vi "Host.vi"() -> ()   [LabVIEW 2019]
uses:
  TypeDef/listChannel.ctl
  ByteGSAPIBase/LimsTestStep/acquisitions.ctl
  <vilib>/Bytelabs/ByteChannelsSetting/ChannelSettingsLib/ChannelsRepos/ChannelsRepoXML/ChannelsRepoXML.lvclass
  C:/Program Files (x86)/National Instruments/LabVIEW 2019/vi.lib/Bytelabs/ByteChannelsSetting/ChannelSettingsLib/ChannelsRepos/ChannelsRepoBase/ChannelsRepoBase.lvclass
  TypeDef/TCPMessage.ctl
  <vilib>/Bytelabs/ByteChannelsSetting/ChannelSettingsLib/ChannelsRepos/ChannelsRepoBase/ChannelsRepoBase.lvclass/ChannelsRepoBase.ctl
  TypeDef/ChannelInfo.ctl
  <vilib>/Bytelabs/ByteChannelsSetting/ChannelSettingsLib/ChannelsClasses/ChannelAnalog/AnalogIn/AnalogIn.lvclass
  ByteGSAPIBase/UpdateChannelsList/fields.ctl
  ByteGSAPIBase/TypeDef/Step.ctl
  ByteGSAPIBase/TypeDef/Asset.ctl
  bytetcp/TCPLib/TCP_Class/TCP.lvclass
  <vilib>/Bytelabs/ByteChannelsSetting/ChannelSettingsLib/ChannelsClasses/ChannelBase/ChannelBase.lvclass
  <vilib>/Bytelabs/ByteChannelsSetting/ChannelSettingsLib/ChannelsRepos/ChannelsRepoBase/ChannelsRepoBase.lvclass
  ByteGSAPIBase/ByteGSAPIBase.lvclass
panel:
  in  "Test":T1={"Step Id"=43, "Test Slug"="T0023", "Duration Seconds"=0.0, "Continous?"=FALSE}
  out "error out":errorcluster
  in  "Stop":bool
  out "Results":T2
  in  "Stop Sequence":bool
  out "Status":string
  out "Raws Readings":cluster{"tag":string, "Value":dbl}[](array[cluster])
  in  "Step  Request":bool
  in  "Channel List":T3[](array[typedef])
  in  "Load":bool
  in  "Configuration":bool
  out "Connected?":bool
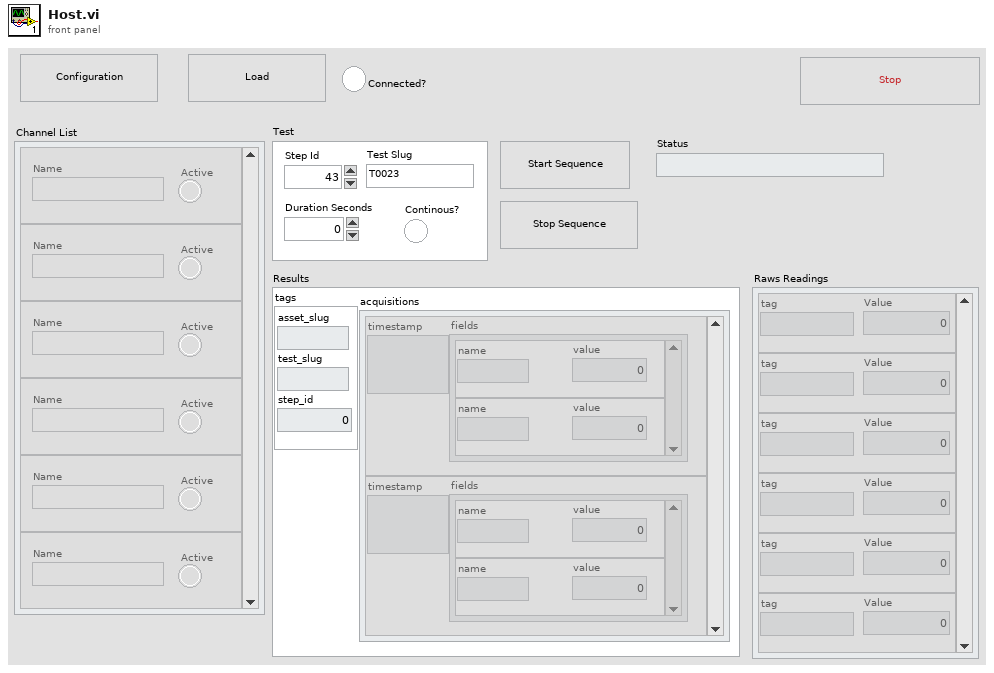
[diagram p1: front panel]
types:
  T1 = cluster{"Step Id":u32, "Test Slug":string, "Duration Seconds":dbl, "Continous?":bool}
  T2 = typedef "ByteGSWebAPI.lvlib/ByteGSAPIBase.lvclass/acquisitions.ctl" = cluster{"tags":cluster{"step_id":i32, "test_slug":string, "asset_slug":string}, "acquisitions":cluster{"timestamp":string, "fields":cluster{"name":string, "value":dbl}[]}[]}
  T3 = typedef "listChannel.ctl" = cluster{"Name":string, "Active":bool}
  T4 = typedef "TCPMessage.ctl" = cluster{"Message":string, "Data":variant}
  T5 = cluster{"Event Registration Refnum":refnum<event-registration>, "ChannelsRepoBase out":refnum<class "ChannelsRepoXML.lvclass">, "TCP_Class":refnum<class "TCP.lvclass">, "Data":variant, "Stauts":string, "notifier out":refnum<notifier>}
  T6 = typedef "ChannelInfo.ctl" = cluster{"Tag":string, "HW Resource":string, "Raw":dbl}
  T7 = typedef "ByteGSWebAPI.lvlib/ByteGSAPIBase.lvclass/fields.ctl" = cluster{"asset_slug":string, "fields":string[]}
  T8 = cluster{"Channel List":T3[], "Test":cluster{"Step Id":u32, "Test Slug":string, "Duration Seconds":dbl, "Continous?":bool}}
  T9 = map{i32, map{string, refnum<class "ChannelBase.lvclass">}}
  T10 = typedef "ByteGSWebAPI.lvlib/ByteGSAPIBase.lvclass/Step.ctl" = cluster{"id":i32, "descrizione":string, "prova":cluster{"slug":string}, "assets":T11[], "criterio_accettazione":string, "valore_criterio_accettazione_max":dbl, "valore_criterio_accettazione_min":dbl, "udm_criterio_accettazione":string, "duration_prova":string, "udm_duration_prova":string, "valore_prova":dbl, "ordine":i32, "user":i32, "link_automation":string, "instruction_automation":string, "data_completamento_checklist":timestamp, "outcome":bool, "step_type":string, "channels":string[]}
  T11 = typedef "ByteGSWebAPI.lvlib/ByteGSAPIBase.lvclass/Asset.ctl" = cluster{"descrizione":string, "slug":string, "id":i32}
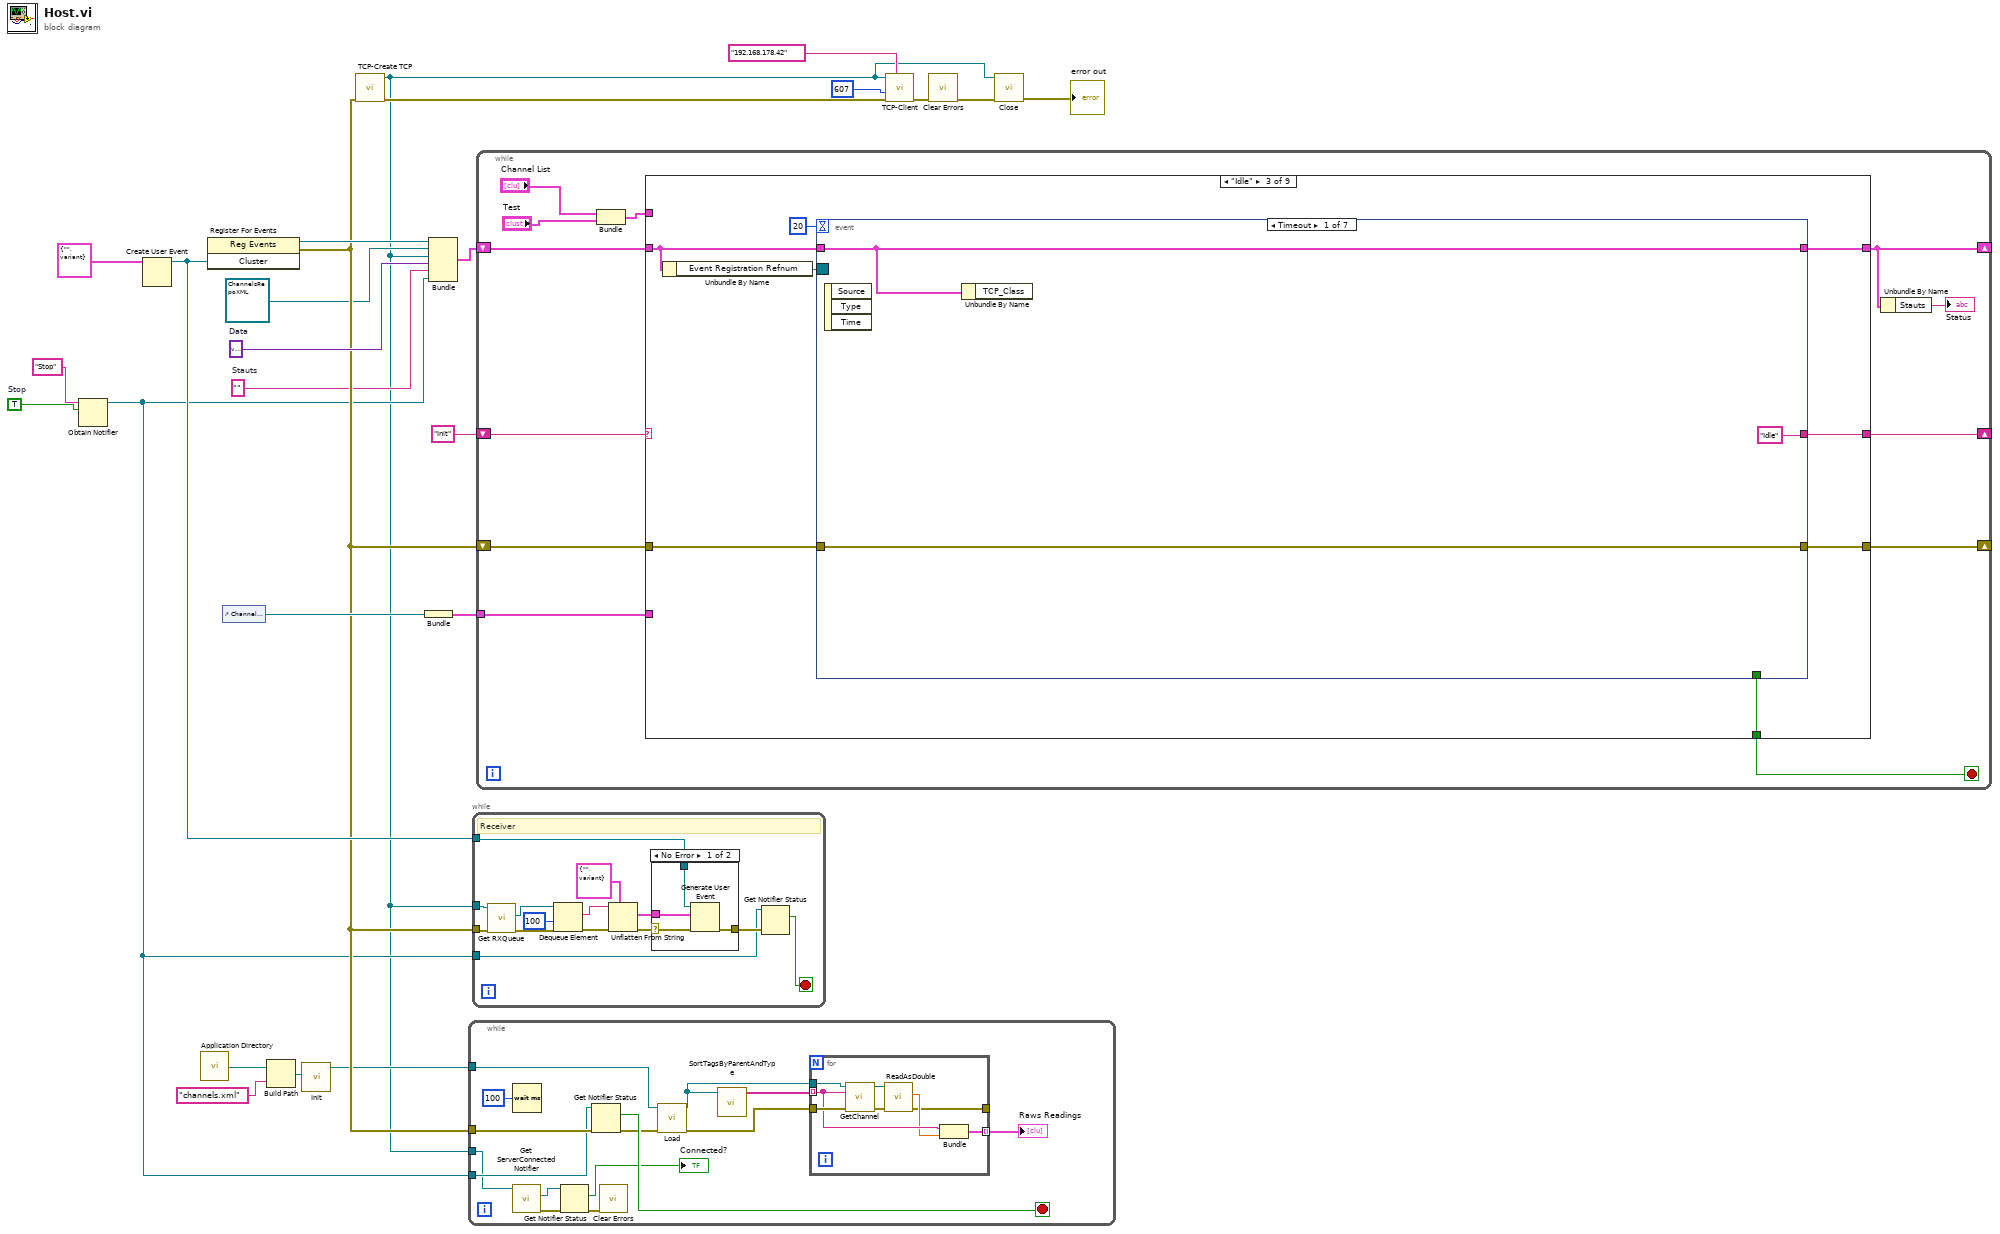
[diagram p0: block diagram]
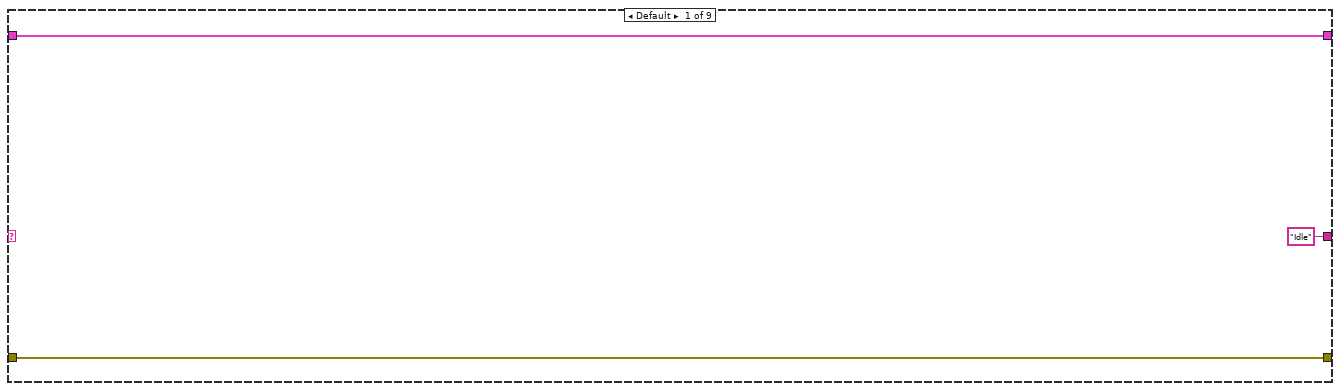
[diagram p2: hidden frame]
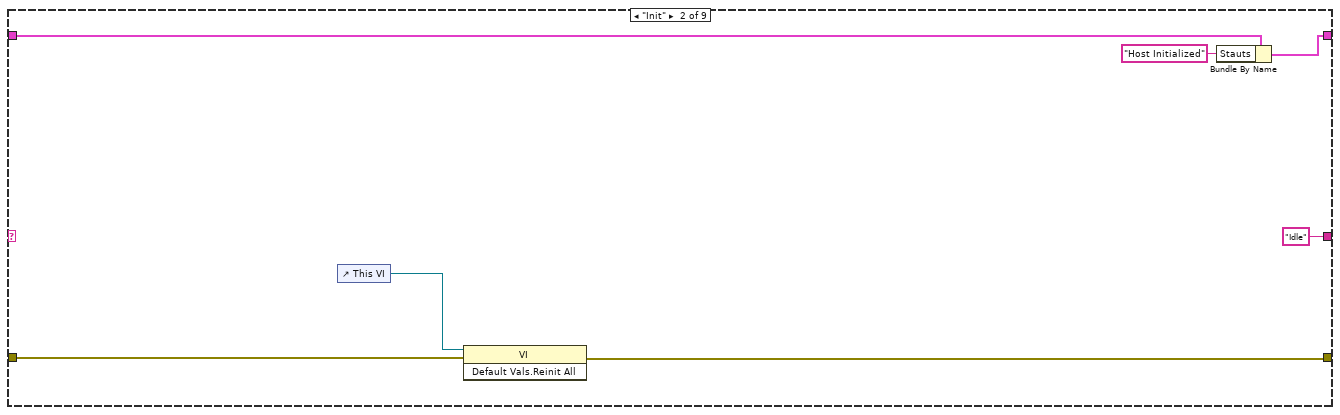
[diagram p3: hidden frame]
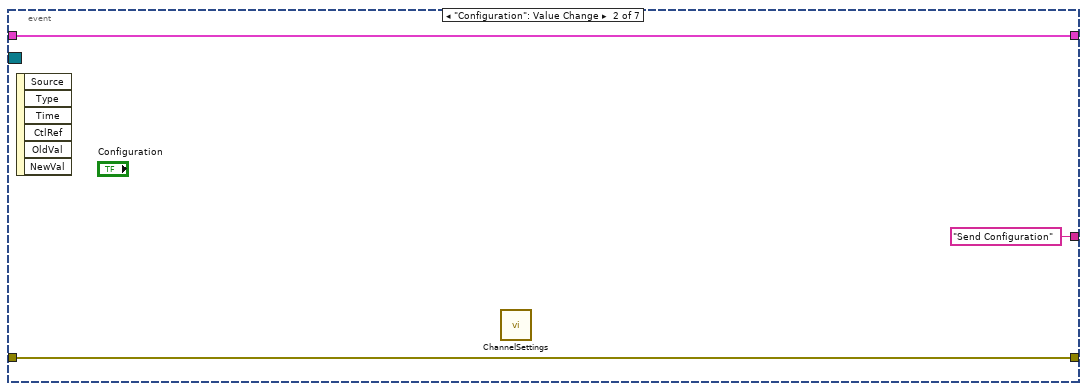
[diagram p4: hidden frame]
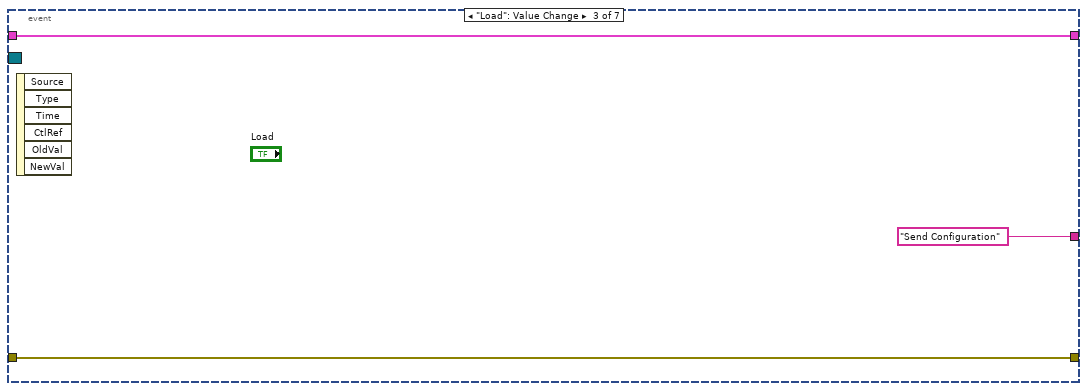
[diagram p5: hidden frame]
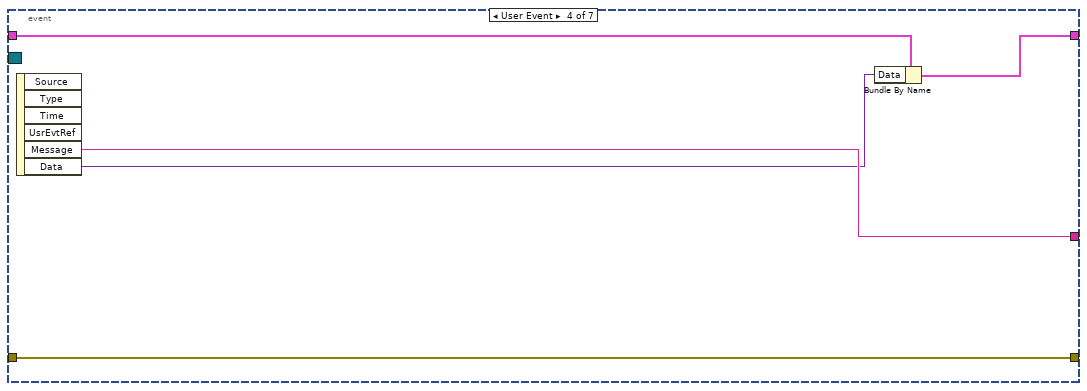
[diagram p6: hidden frame]
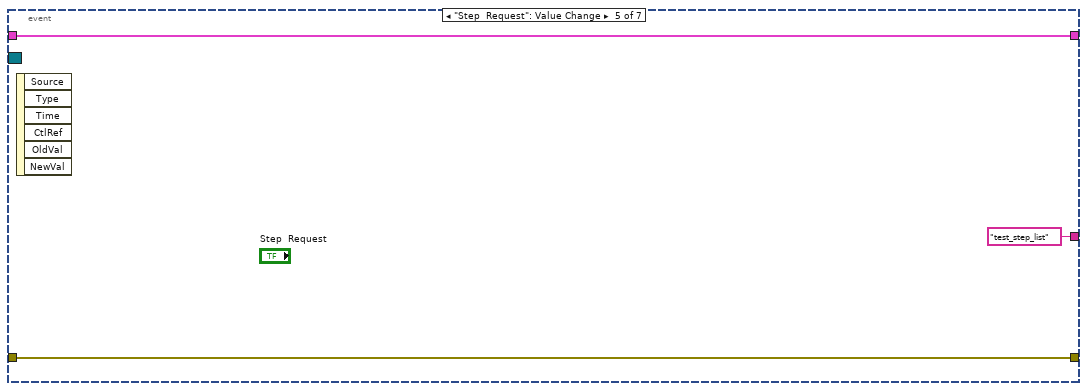
[diagram p7: hidden frame]
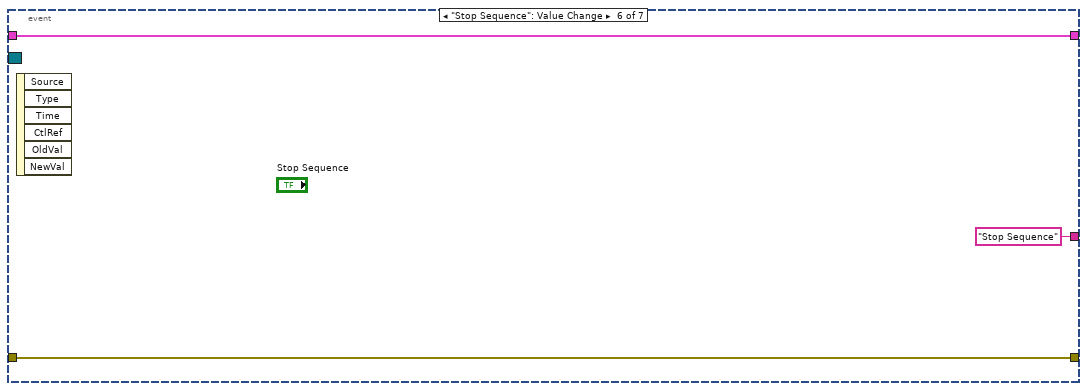
[diagram p8: hidden frame]
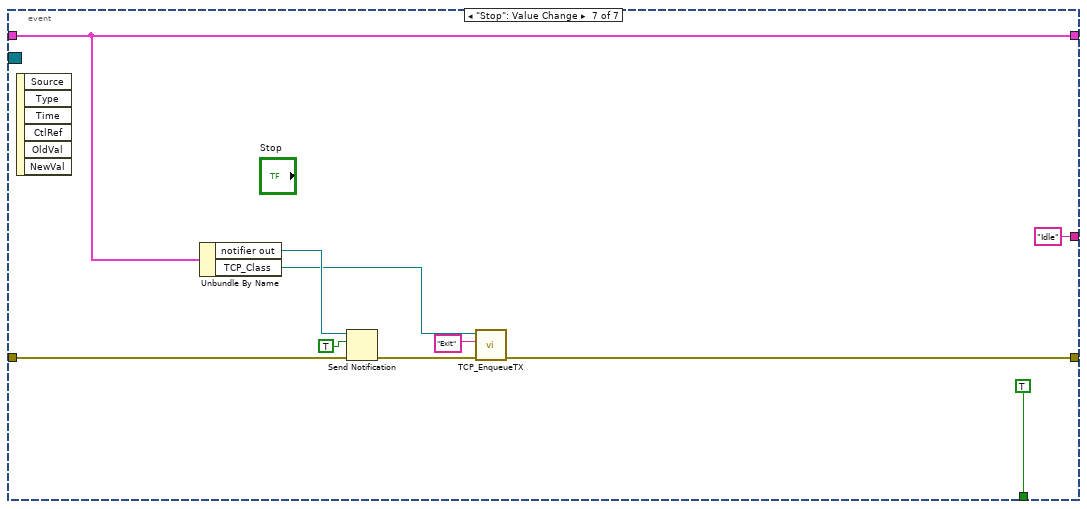
[diagram p9: hidden frame]
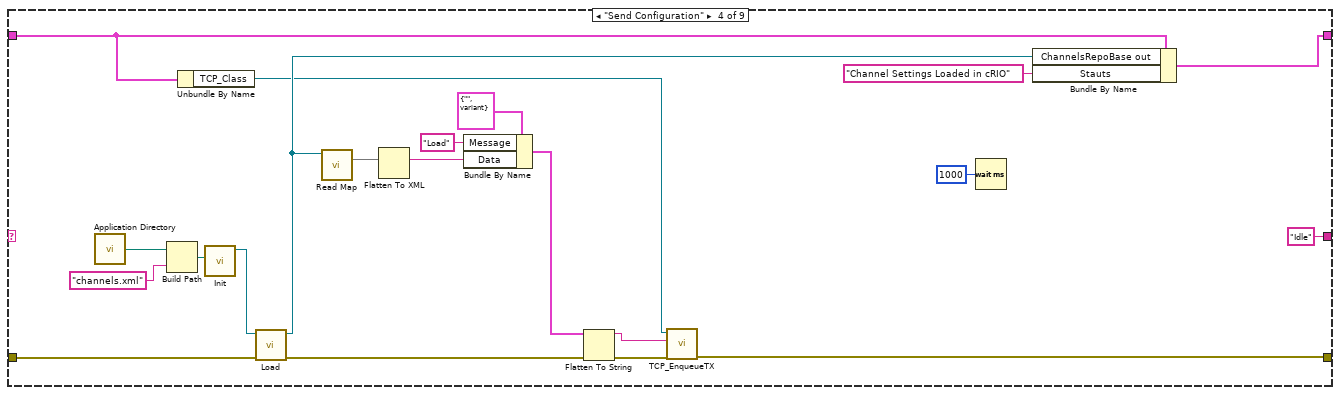
[diagram p10: hidden frame]
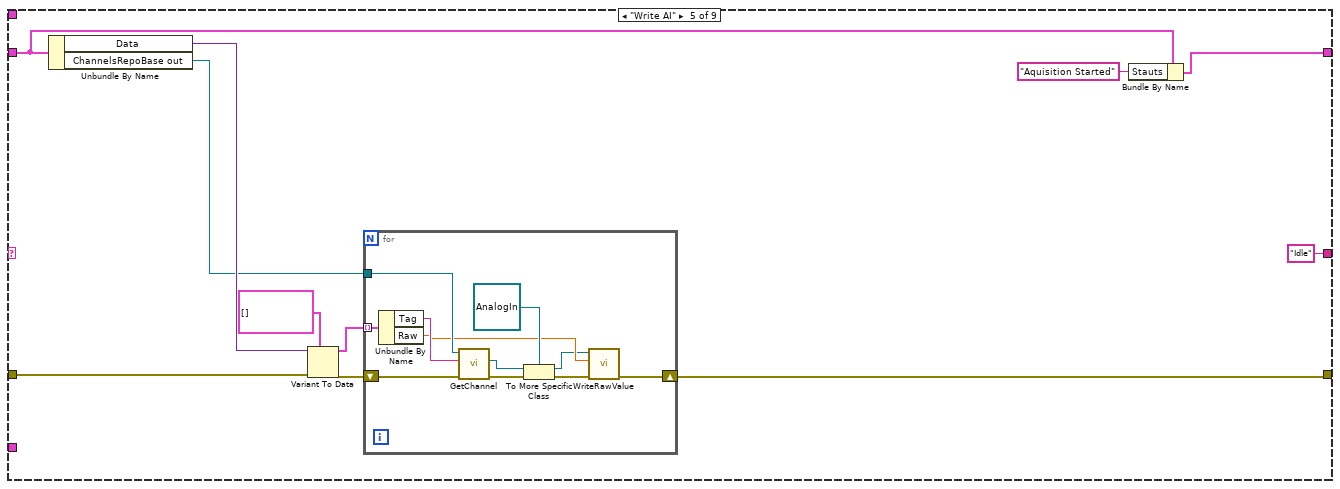
[diagram p11: hidden frame]
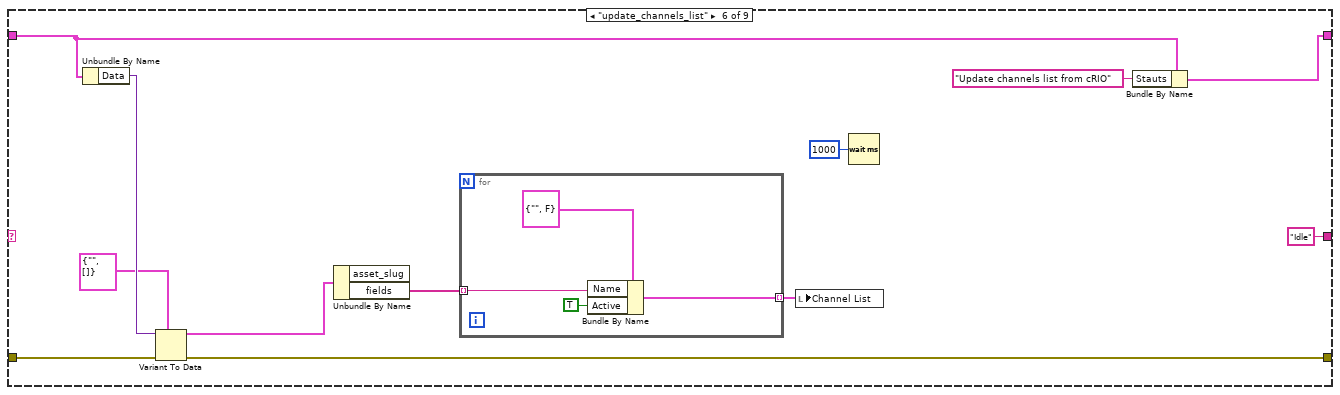
[diagram p12: hidden frame]
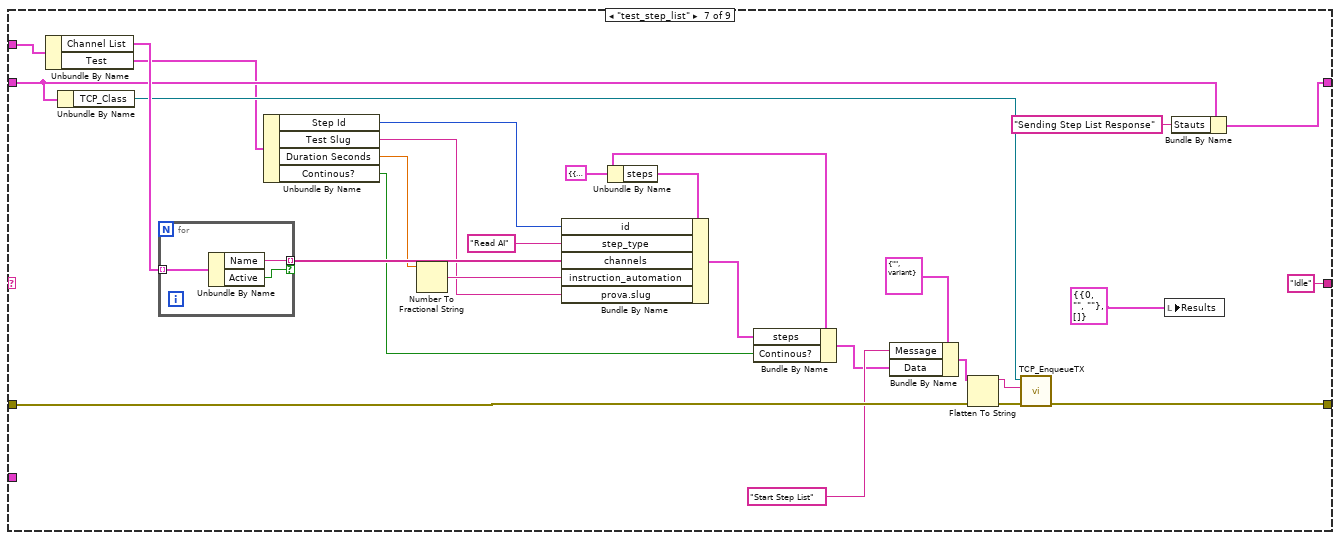
[diagram p13: hidden frame]
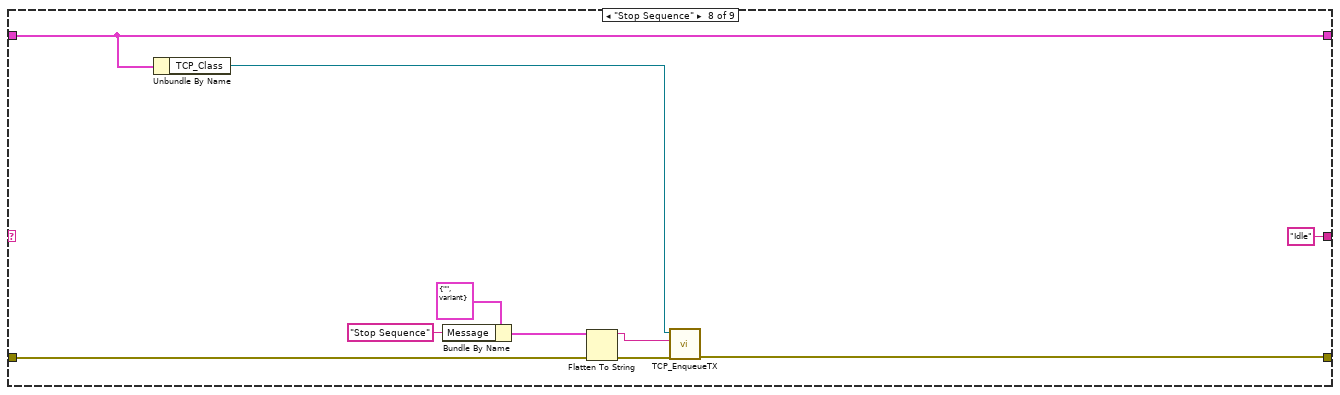
[diagram p14: hidden frame]
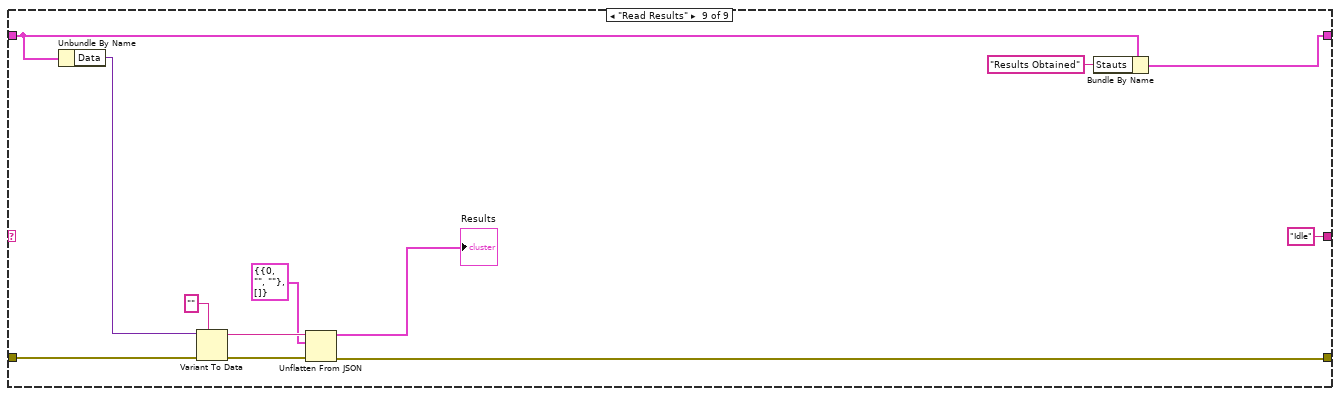
[diagram p15: hidden frame]
diagram:
  w11 = TRUE  # Stop
  w12 = ""  # Stauts
  w17 = variant  # Data
  n1 = Obtain Notifier(name (unnamed)="Stop", notification data type=w11) -> (notifier out=w9:refnum<notifier>)  [unwired: 2 in, 2 out]
  n2 = Create User Event(user event datatype=T4 {"Message"="", "Data"=variant} ("Cluster")) -> (user event=w22:refnum<user-event>)  [unwired: 1 in, 1 out]
  n3 = call <vilib>:"Application Directory.vi"() -> ("Application Directory"=w4:path)
  n4 = register-events(w22) -> (reference out=w21:refnum<event-registration>, error out=w14:errorcluster)  [unwired: 2 in]
  n5 = control-ref of="Channel List"() -> (w16:refnum<vi>)
  n6 = Build Path(base path=w4, name or relative path="channels.xml") -> (appended path=w5:path)
  n7 = call <vilib>:"Init.vi"("XML file path"=w5) -> ("ChannelsRepoXML out"=w2:refnum<class "ChannelsRepoXML.lvclass">)  [unwired: 10 in]
  n8 = call "TCP-Create TCP.vi"("error in (no error)"=w14) -> ("error out"=w23:errorcluster, "TCP_Class"=w1:refnum<class "TCP.lvclass">)  [unwired: 8 in, 1 out]
  n9 = Bundle("Channel List"=w16) -> (w15:cluster{"Channel List":refnum<vi>})  [unwired: 1 in]
  n10 = Bundle("Event Registration Refnum"=w21, "ChannelsRepoBase out"=refnum<class "ChannelsRepoXML.lvclass"> refnum, "TCP_Class"=w1, "Data"=w17, "Stauts"=w12, "notifier out"=w9) -> (w20:T5)  [unwired: 1 in]
  n11 = while {
    tunnel: w14 -> [w36]
    tunnel: w9 -> [w35]
    tunnel: w2 -> [w32]
    tunnel: w1 -> [w27]
    stop <- w34 stop-if-true
    n12 = call-dynamic "Get ServerConnectedNotifier.vi"("TCP in"=w27) -> ("error out"=w29:errorcluster, "IsServerConnected?"=w28:refnum<notifier>)  [unwired: 8 in, 1 out]
    n13 = Wait (ms)(milliseconds to wait=u32 100) -> ()  [unwired: 1 out]
    n14 = Get Notifier Status(notifier=w28, error in (no error)=w29) -> (current notification=→"Connected?":bool, error out=w30:errorcluster)  [unwired: 3 out]
    n15 = Get Notifier Status(notifier=w35, error in (no error)=w36) -> (current notification=w34:bool, error out=w33:errorcluster)  [unwired: 3 out]
    n16 = call <vilib>:"Clear Errors.vi"("error in (no error)"=w30) -> ()  [unwired: 5 in, 2 out]
    n17 = call <vilib>:"Load.vi"("error in (no error)"=w33, "ChannelsRepoBase in"=w32) -> ("error out"=w38:errorcluster, "ChannelsRepoBase out"=w37:refnum<class "ChannelsRepoXML.lvclass">)  [unwired: 7 in, 1 out]
    n18 = call <vilib>:"SortTagsByParentAndType.vi"("ChannelsRepoBase in"=w37) -> ("sorted tags"=w40:string[])  [unwired: 8 in, 2 out]
    n19 = for {
      tunnel: w38 -> [w48]
      tunnel: w40 -> [w45] mode=indexing
      tunnel: [w43] -> w39 mode=indexing
      tunnel: [w42] -> _
      tunnel: w37 -> [w41]
      n20 = call <vilib>:"GetChannel.vi"("error in (no error)"=w48, "tag"=w45, "ChannelsRepoBase in"=w41) -> ("error out"=w47:errorcluster, "channel"=w46:refnum<class "ChannelBase.lvclass">)  [unwired: 5 in, 2 out]
      n21 = call-dynamic "ReadAsDouble.vi"("error in (no error)"=w47, "ChannelBase in"=w46) -> ("error out"=w42:errorcluster, "Value"=w44:dbl)  [unwired: 7 in, 1 out]
      n22 = Bundle("tag"=w45, "Value"=w44) -> (w43:cluster{"tag":string, "Value":dbl})  [unwired: 1 in]
    }
    "Raws Readings" <- w39
  }
  n23 = while {
    tunnel: w1 -> [w57]
    tunnel: w14 -> [w58]
    tunnel: w22 -> [w61]
    tunnel: w9 -> [w51]
    stop <- w50 stop-if-true
    # "Receiver"
    n24 = call-dynamic "Get RXQueue.vi"("error in (no error)"=w58, "TCP in"=w57) -> ("error out"=w56:errorcluster, "RX"=w53:refnum<queue>)  [unwired: 7 in, 1 out]
    n25 = Dequeue Element(queue=w53, timeout in ms (-1)=100, error in (no error)=w56) -> (element=w54:string, error out=w55:errorcluster)  [unwired: 2 out]
    n26 = Unflatten From String(type=T4 {"Message"="", "Data"=variant} ("Cluster"), binary string=w54, error in (no error)=w55) -> (value=w60:T4, error out=w62:errorcluster)  [unwired: 2 in, 1 out]
    n27 = case shown="No Error" w62 {
      selector: w62 -> [w66 _]
      tunnel: w61 -> [w65 _]
      tunnel: w60 -> [w64 _]
      tunnel: [w63 _] -> w52
      frame No Error {
        n28 = Generate User Event(user event=w65, event data cluster=w64, error in=w66) -> (error out=w63:errorcluster)  [unwired: 1 in, 1 out]
      }
      frame Error {
      }
    }
    n29 = Get Notifier Status(notifier=w51, error in (no error)=w52) -> (current notification=w50:bool)  [unwired: 4 out]
  }
  n30 = while {
    shift-right: [w70] -> _
    shift-left: w20 -> [w76]
    shift-right: [w77] -> _
    shift-left: "Init" -> [w78]
    shift-right: [w74] -> _
    shift-left: w14 -> [w75]
    tunnel: w15 -> [w71]
    stop <- w68 stop-if-true
    n31 = Bundle("Channel List"="Channel List", "Test"="Test") -> (w72:T8)  [unwired: 1 in]
    n32 = case shown="\"Idle\"" w78 {
      tunnel: ["Idle" "Idle" w93 "Idle" "Idle" ("Message") "Idle" ("Message") "Idle" ("Message") "Idle" ("Message") "Idle" ("Message")] -> w77
      tunnel: w76 -> [w81 w84 w91 w135 w150 w174 w199 w217 w230]
      tunnel: [w81 w82 w92 w134 w149 w172 w198 w217 w228] -> w70
      tunnel: w75 -> [w79 w87 w95 w137 w153 w181 w212 w220 w234]
      tunnel: [w79 w85 w94 w131 w152 w176 w202 w219 w233] -> w74
      tunnel: w72 -> [_ _ _ _ _ _ w210 _ _]
      tunnel: w71 -> [_ _ _ _ _ _ _ _ _]
      tunnel: [_ _ w89 _ _ _ _ _ _] -> w68
      frame Default {
      }
      frame "Init" {
        n33 = control-ref of="This VI"() -> (w86:refnum<vi>)
        n34 = invoke class="VI" method="Default Vals.Reinit All"(reference=w86, error in=w87) -> (error out=w85:errorcluster)  [unwired: 1 in, 2 out]
        n35 = Bundle By Name(cluster=w84, "Stauts"="Host Initialized") -> (w82:T5)
      }
      frame "Idle" {
        n36 = Unbundle By Name(w91) -> ("Event Registration Refnum"=w90:refnum<event-registration>)
        n37 = event shown="[0] Timeout" {
          selector: w90 -> [_ _ _ _ _ _ _]
          dyn-events: _ -> [_ _ _ _ _ _ _]
          timeout: 20 -> [_ _ _ _ _ _ _]
          tunnel: w91 -> [w98 w102 w105 w109 w113 w115 w124]
          tunnel: w95 -> [w97 w101 w103 w106 w112 w116 w122]
          tunnel: [w97 w101 w103 w106 w112 w116 w119] -> w94
          tunnel: ["Idle" "Send Configuration" "Send Configuration" w110 "test_step_list" ("Message") "Stop Sequence" ("Message") "Idle" ("Message")] -> w93
          tunnel: [w98 w102 w105 w108 w113 w115 w124] -> w92
          tunnel: [_ _ _ _ _ _ TRUE] -> w89
          event Timeout {
            n38 = event-data() -> ()  [unwired: 1 in, 3 out]
            n39 = Unbundle By Name(w98) -> ()  [unwired: 1 out]
          }
          event "Configuration": Value Change {
            n40 = event-data() -> ()  [unwired: 1 in, 6 out]
            n41 = call "ChannelSettings.vi"() -> ()  [unwired: 12 in]
          }
          event "Load": Value Change {
            n42 = event-data() -> ()  [unwired: 1 in, 6 out]
          }
          event User Event {
            n43 = event-data() -> ("Message"=w110:string, "Data"=w107:variant)  [unwired: 1 in, 4 out]
            n44 = Bundle By Name(cluster=w109, "Data"=w107) -> (w108:T5)
          }
          event "Step  Request": Value Change {
            n45 = event-data() -> ()  [unwired: 1 in, 6 out]
          }
          event "Stop Sequence": Value Change {
            n46 = event-data() -> ()  [unwired: 1 in, 6 out]
          }
          event "Stop": Value Change {
            n47 = event-data() -> ()  [unwired: 1 in, 6 out]
            n48 = Unbundle By Name(w124) -> ("notifier out"=w123:refnum<notifier>, "TCP_Class"=w118:refnum<class "TCP.lvclass">)
            n49 = Send Notification(notification=TRUE, notifier=w123, error in (no error)=w122) -> (error out=w120:errorcluster)  [unwired: 1 out]
            n50 = call-dynamic "TCP_EnqueueTX.vi"("error in (no error)"=w120, "Msg to Transmit"="Exit", "TCP in"=w118) -> ("error out"=w119:errorcluster)  [unwired: 7 in, 1 out]
          }
        }
      }
      frame "Send Configuration" {
        n51 = call <vilib>:"Application Directory.vi"() -> ("Application Directory"=w141:path)
        n52 = Build Path(base path=w141, name or relative path="channels.xml") -> (appended path=w140:path)
        n53 = Unbundle By Name(w135) -> ("TCP_Class"=w130:refnum<class "TCP.lvclass">)
        n54 = call <vilib>:"Init.vi"("XML file path"=w140) -> ("ChannelsRepoXML out"=w139:refnum<class "ChannelsRepoXML.lvclass">)  [unwired: 10 in]
        n55 = call <vilib>:"Load.vi"("error in (no error)"=w137, "ChannelsRepoBase in"=w139) -> ("error out"=w136:errorcluster, "ChannelsRepoBase out"=w133:refnum<class "ChannelsRepoXML.lvclass">)  [unwired: 7 in, 1 out]
        n56 = call <vilib>:"Read Map.vi"("ChannelsRepoBase in"=w133) -> ("Map"=w144:T9)  [unwired: 9 in, 1 out]
        n57 = Flatten To XML(anything=w144) -> (xml string=w143:string)
        n58 = Bundle By Name(cluster=T4 {"Message"="", "Data"=variant} ("Cluster"), "Message"="Load", "Data"=w143) -> (w142:T4)
        n59 = Flatten To String(anything=w142, error in (no error)=w136) -> (data string=w129:string, error out=w132:errorcluster)  [unwired: 2 in, 1 out]
        n60 = call-dynamic "TCP_EnqueueTX.vi"("error in (no error)"=w132, "Msg to Transmit"=w129, "TCP in"=w130) -> ("error out"=w131:errorcluster)  [unwired: 7 in, 1 out]
        n61 = Wait (ms)(milliseconds to wait=u32 1000) -> ()  [unwired: 1 out]
        n62 = Bundle By Name(cluster=w135, "ChannelsRepoBase out"=w133, "Stauts"="Channel Settings Loaded in cRIO") -> (w134:T5)
      }
      frame "Write AI" {
        n63 = Unbundle By Name(w150) -> ("Data"=w158:variant, "ChannelsRepoBase out"=w155:refnum<class "ChannelsRepoXML.lvclass">)
        n64 = Variant To Data(error in=w153, type=T6[] [] ("Array"), Variant=w158) -> (data=w154:T6[], error out=w156:errorcluster)
        n65 = for {
          tunnel: w155 -> [w167]
          shift-right: [w161] -> w152
          shift-left: w156 -> [w169]
          tunnel: w154 -> [w159] mode=indexing
          n66 = Unbundle By Name(w159) -> ("Tag"=w168:string, "Raw"=w163:dbl)
          n67 = call <vilib>:"GetChannel.vi"("error in (no error)"=w169, "tag"=w168, "ChannelsRepoBase in"=w167) -> ("error out"=w166:errorcluster, "channel"=w160:refnum<class "ChannelBase.lvclass">)  [unwired: 5 in, 2 out]
          n68 = To More Specific Class(target class=refnum<class "AnalogIn.lvclass"> refnum ("ChannelSettings.lvlib:ChannelsClasses.lvlib:AnalogIn.lvclass"), reference=w160, error in=w166) -> (specific class reference=w162:refnum<class "AnalogIn.lvclass">, error out=w164:errorcluster)
          n69 = call <vilib>:"WriteRawValue.vi"("error in (no error)"=w164, "Raw value"=w163, "AnalogIn in"=w162) -> ("error out"=w161:errorcluster)  [unwired: 7 in, 1 out]
        }
        n70 = Bundle By Name(cluster=w150, "Stauts"="Aquisition Started") -> (w149:T5)
      }
      frame "update_channels_list" {
        n71 = Unbundle By Name(w174) -> ("Data"=w180:variant)
        n72 = Variant To Data(error in=w181, type=T7 {"asset_slug"="", "fields"=[]} ("Channels"), Variant=w180) -> (data=w175:T7, error out=w176:errorcluster)
        n73 = Unbundle By Name(w175) -> ("fields"=w178:string[])  [unwired: 1 out]
        n74 = for {
          tunnel: w178 -> [w184] mode=indexing
          tunnel: [w182] -> w177 mode=indexing
          n75 = Bundle By Name(cluster=T3 {"Name"="", "Active"=FALSE} ("Cluster"), "Name"=w184, "Active"=TRUE) -> (w182:T3)
        }
        n76 = local write "Channel List"(w177) -> ()
        n77 = Wait (ms)(milliseconds to wait=u32 1000) -> ()  [unwired: 1 out]
        n78 = Bundle By Name(cluster=w174, "Stauts"="Update channels list from cRIO") -> (w172:T5)
      }
      frame "test_step_list" {
        w189 = cluster{"steps":T10, "Continous?":bool} {"steps"={"id"=0, "descrizione"="", "prova"={"slug"=""}, "assets"=[], "criterio_accettazione"="", "valore_criterio_accettazione_max"=0.0, "valore_criterio_accettazione_min"=0.0, "udm_criterio_accettazione"="", "duration_prova"="", "udm_duration_prova"="", "valore_prova"=0.0, "ordine"=0, "user"=0, "link_automation"="", "instruction_automation"="", "data_completamento_checklist"=timestamp(0 s since 1904-01-01), "outcome"=FALSE, "step_type"="", "channels"=[]}, "Continous?"=FALSE}
        n79 = Unbundle By Name(w210) -> ("Channel List"=w209:T3[], "Test"=w192:T1)
        n80 = Unbundle By Name(w199) -> ("TCP_Class"=w201:refnum<class "TCP.lvclass">)
        n81 = for {
          tunnel: w209 -> [w215] mode=indexing
          tunnel: [w214] -> w208 mode=indexing if=w213
          n82 = Unbundle By Name(w215) -> ("Name"=w214:string, "Active"=w213:bool)
        }
        n83 = Unbundle By Name(w192) -> ("Step Id"=w194:u32, "Test Slug"=w193:string, "Duration Seconds"=w191:dbl, "Continous?"=w187:bool)
        n84 = Number To Fractional String(number=w191) -> (F-format string=w196:string)  [unwired: 3 in]
        n85 = Unbundle By Name(w189) -> ("steps"=w190:T10)
        n86 = Bundle By Name(cluster=w190, "id"=w194, "step_type"="Read AI", "channels"=w208, "instruction_automation"=w196, "prova.slug"=w193) -> (w188:T10)
        n87 = Bundle By Name(cluster=w189, "steps"=w188, "Continous?"=w187) -> (w186:cluster{"steps":T10, "Continous?":bool})
        n88 = Bundle By Name(cluster=T4 {"Message"="", "Data"=variant} ("Cluster"), "Message"="Start Step List", "Data"=w186) -> (w204:T4)
        n89 = Flatten To String(anything=w204, error in (no error)=w212) -> (data string=w203:string, error out=w205:errorcluster)  [unwired: 2 in, 1 out]
        n90 = call-dynamic "TCP_EnqueueTX.vi"("error in (no error)"=w205, "Msg to Transmit"=w203, "TCP in"=w201) -> ("error out"=w202:errorcluster)  [unwired: 7 in, 1 out]
        n91 = local write "Results"(T2 {"tags"={"step_id"=0, "test_slug"="", "asset_slug"=""}, "acquisitions"=[]}) -> ()
        n92 = Bundle By Name(cluster=w199, "Stauts"="Sending Step List Response") -> (w198:T5)
      }
      frame "Stop Sequence" {
        n93 = Unbundle By Name(w217) -> ("TCP_Class"=w216:refnum<class "TCP.lvclass">)
        n94 = Bundle By Name(cluster=T4 {"Message"="", "Data"=variant} ("Cluster"), "Message"="Stop Sequence") -> (w223:T4)
        n95 = Flatten To String(anything=w223, error in (no error)=w220) -> (data string=w221:string, error out=w222:errorcluster)  [unwired: 2 in, 1 out]
        n96 = call-dynamic "TCP_EnqueueTX.vi"("error in (no error)"=w222, "Msg to Transmit"=w221, "TCP in"=w216) -> ("error out"=w219:errorcluster)  [unwired: 7 in, 1 out]
      }
      frame "Read Results" {
        n97 = Unbundle By Name(w230) -> ("Data"=w232:variant)
        n98 = Variant To Data(error in=w234, type="", Variant=w232) -> (data=w235:string, error out=w237:errorcluster)
        n99 = Unflatten From JSON(JSON string=w235, type and defaults=T2 {"tags"={"step_id"=0, "test_slug"="", "asset_slug"=""}, "acquisitions"=[]}, error in (no error)=w237) -> (value=→"Results":T2, error out=w233:errorcluster)  [unwired: 4 in]
        n100 = Bundle By Name(cluster=w230, "Stauts"="Results Obtained") -> (w228:T5)
      }
    }
    n101 = Unbundle By Name(w70) -> ("Stauts"=→"Status":string)
  }
  n102 = call "TCP-Client.vi"("IP address"="192.168.178.42", "error in (no error)"=w23, "TXport"=u16 607 ("port"), "TCP.lvclass"=w1) -> ("error out"=w7:errorcluster)  [unwired: 7 in]
  n103 = call <vilib>:"Clear Errors.vi"("error in (no error)"=w7) -> ("error out"=w6:errorcluster)  [unwired: 5 in, 1 out]
  n104 = call-dynamic "Close.vi"("error in (no error)"=w6, "TCP in"=w1) -> ("error out"=→"error out":errorcluster)  [unwired: 5 in, 4 out]
